vi "rcpacini_m_merge_icon.vi"(6 "Variant in":variant, 7 "Shift Pressed?":bool, 8 "error in (no error)":errorcluster, 10 "QD Combo Box Ref":refnum<vi>, 11 "QD Launch VI Ref":refnum<vi>) -> (0 "error out":errorcluster, 4 "Variant out":variant)   [LabVIEW 2019]
doc: "Merge all icon layers to minimize space and avoid layer template collisions.\n\nCreated by: Ryan Pacini\n\nDefault Shortcut - [M]"
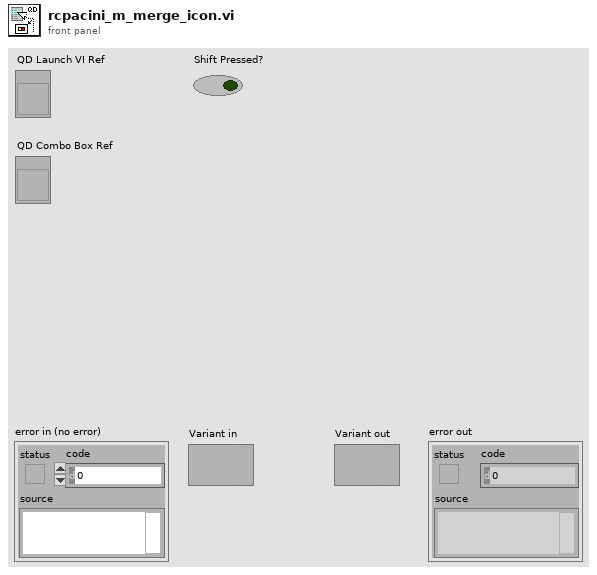
[diagram p1: front panel]
types:
  T1 = typedef "imagedata.ctl" = cluster{"image type":i32, "image depth":i32, "image":u8[], "mask":u8[], "colors":u32[], "Rectangle":cluster{"left":i16, "top":i16, "right":i16, "bottom":i16}}
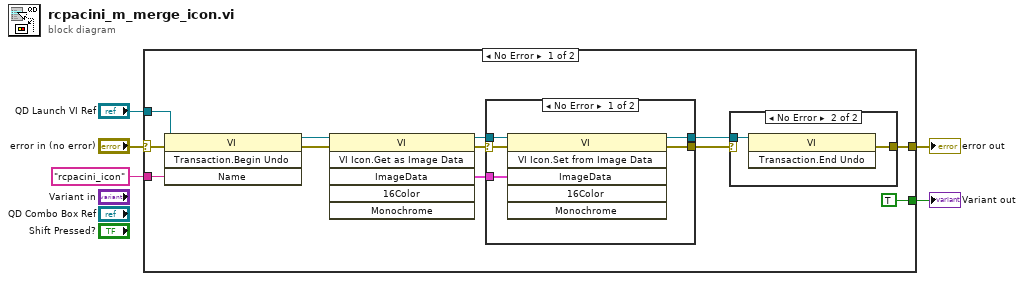
[diagram p0: block diagram]
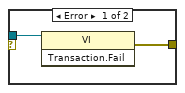
[diagram p3: hidden frame]
diagram:
  n1 = case shown="No Error" "error in (no error)" {
    selector: "error in (no error)" -> [w17 w29]
    tunnel: [w16 w29] -> w1
    tunnel: "QD Launch VI Ref" -> [w13 _]
    tunnel: "rcpacini_icon" ("Undo Name") -> [w15 _]
    tunnel: [TRUE _] -> w2
    frame No Error {
      n2 = invoke class="VI" method="Transaction.Begin Undo"(reference=w13, error in=w17, "Name"=w15) -> (reference out=w8:refnum<vi>, error out=w9:errorcluster)  [unwired: 1 in, 2 out]
      n3 = invoke class="VI" method="VI Icon.Get as Image Data"(reference=w8, error in=w9) -> (reference out=w12:refnum<vi>, error out=w10:errorcluster, "ImageData"=w11:T1)  [unwired: 4 in, 3 out]
      n4 = case shown="No Error" w10 {
        selector: w10 -> [w20 w24]
        tunnel: w12 -> [w22 w23]
        tunnel: w11 -> [w21 _]
        tunnel: [w19 w24] -> w7
        tunnel: [w18 w23] -> w6
        frame No Error {
          n5 = invoke class="VI" method="VI Icon.Set from Image Data"(reference=w22, error in=w20, "ImageData"=w21) -> (reference out=w18:refnum<vi>, error out=w19:errorcluster)  [unwired: 3 in, 4 out]
        }
        frame Error {
        }
      }
      n6 = case shown="No Error" w7 {
        tunnel: w6 -> [w25 w27]
        tunnel: [w26 w28] -> w16
        frame Error {
          n7 = invoke class="VI" method="Transaction.Fail"(reference=w25) -> (error out=w26:errorcluster)  [unwired: 2 in, 2 out]
        }
        frame No Error {
          n8 = invoke class="VI" method="Transaction.End Undo"(reference=w27) -> (error out=w28:errorcluster)  [unwired: 2 in, 2 out]
        }
      }
    }
    frame Error {
    }
  }
  "error out" <- w1
  "Variant out" <- w2
